vi "LOGclose.vi"(8 "error in (no error)":errorcluster) -> ()   [LabVIEW 2025, in "LOGlib.lvlib"]
uses:
  LOGlib.lvlib
  <vilib>/Field R&D Services/Logger/Field_RnD_Services_Logger_Toolkit.lvlib
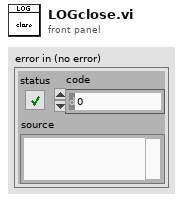
[diagram p1: front panel]
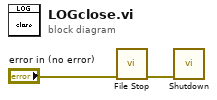
[diagram p0: block diagram]
diagram:
  n1 = call <vilib>:"File Stop.vi"("Error In"="error in (no error)") -> ("Error Out"=w2:errorcluster)  [unwired: 10 in]
  n2 = call <vilib>:"Shutdown.vi"("Error In"=w2) -> ()  [unwired: 10 in, 1 out]
